vi "Step SSO.vi"(11 "Step Actuator Values In":T1) -> ()   [LabVIEW 2014]
uses:
  Step Deployment Actuator Values.ctl
  <vilib>/Rock Robotics/WPI/Solenoid/WPI_SolenoidValue.ctl
  Global Variables/Refnum Names.vi
  <vilib>/Rock Robotics/WPI/Solenoid/WPI_SolenoidSetEnum.vi
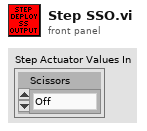
[diagram p1: front panel]
types:
  T1 = typedef "Step Deployment Actuator Values.ctl" = cluster{"Scissors":T2}
  T2 = typedef "WPI_SolenoidValue.ctl" = enum16{"Off", "On", "Forward", "Reverse"}
  T3 = typedef "WPI_SolenoidDevRef.ctl" = cluster{"DevStatus":errorcluster, "Pneumatics Control Module":u8, "Forward Solenoid Channel":T4, "Reverse Solenoid Channel":T4}
  T4 = typedef "WPI_SolenoidChannel.ctl" = enum8{"Solenoid 0", "Solenoid 1", "Solenoid 2", "Solenoid 3", "Solenoid 4", "Solenoid 5", "Solenoid 6", "Solenoid 7", "Invalid"}
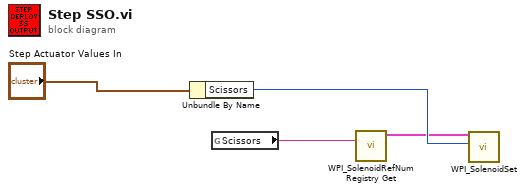
[diagram p0: block diagram]
diagram:
  n1 = Unbundle By Name("Step Actuator Values In") -> ("Scissors"=w3:T2)
  n2 = global read "Refnum Names.vi" "Scissors"() -> (w1:string)
  n3 = call <vilib>:"WPI_SolenoidRefNum Registry Get.vi"("refnum name"=w1) -> ("SolenoidDevRef"=w2:T3)  [unwired: 9 in, 1 out]
  n4 = call-poly <vilib>:"WPI_SolenoidSet.vi"("Value"=w3, "SolenoidDevRef"=w2) -> ()  [unwired: 8 in, 2 out]
